vi "ReadEEPROMtoImage.vi"(8 "error in (no error)":errorcluster, 10 "Automation Refnum":refnum<k7>, 11 "IN":T1={"step name 1"="", "updata 2"="1000", "limitdata 3"="", "load vi name 4"="", "parameter 5"=""}) -> (0 "error out":errorcluster, 2 "reference out":refnum<k7>, 3 "Cluster":T2)   [LabVIEW 2013]
uses:
  Sub vi/Global constant.vi
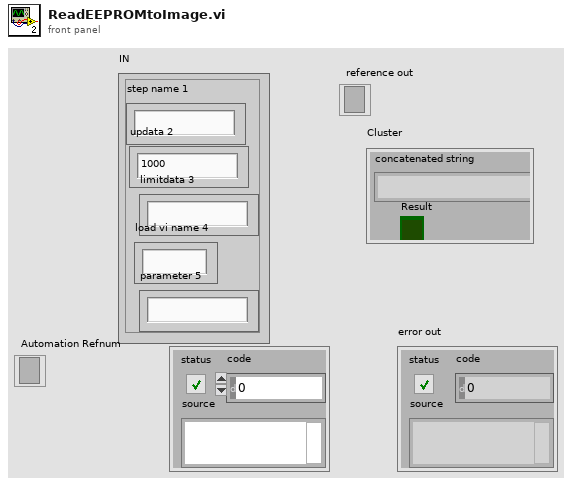
[diagram p1: front panel]
types:
  T1 = cluster{"step name 1":string, "updata 2":string, "limitdata 3":string, "load vi name 4":string, "parameter 5":string}
  T2 = cluster{"concatenated string":string, "Result":bool}
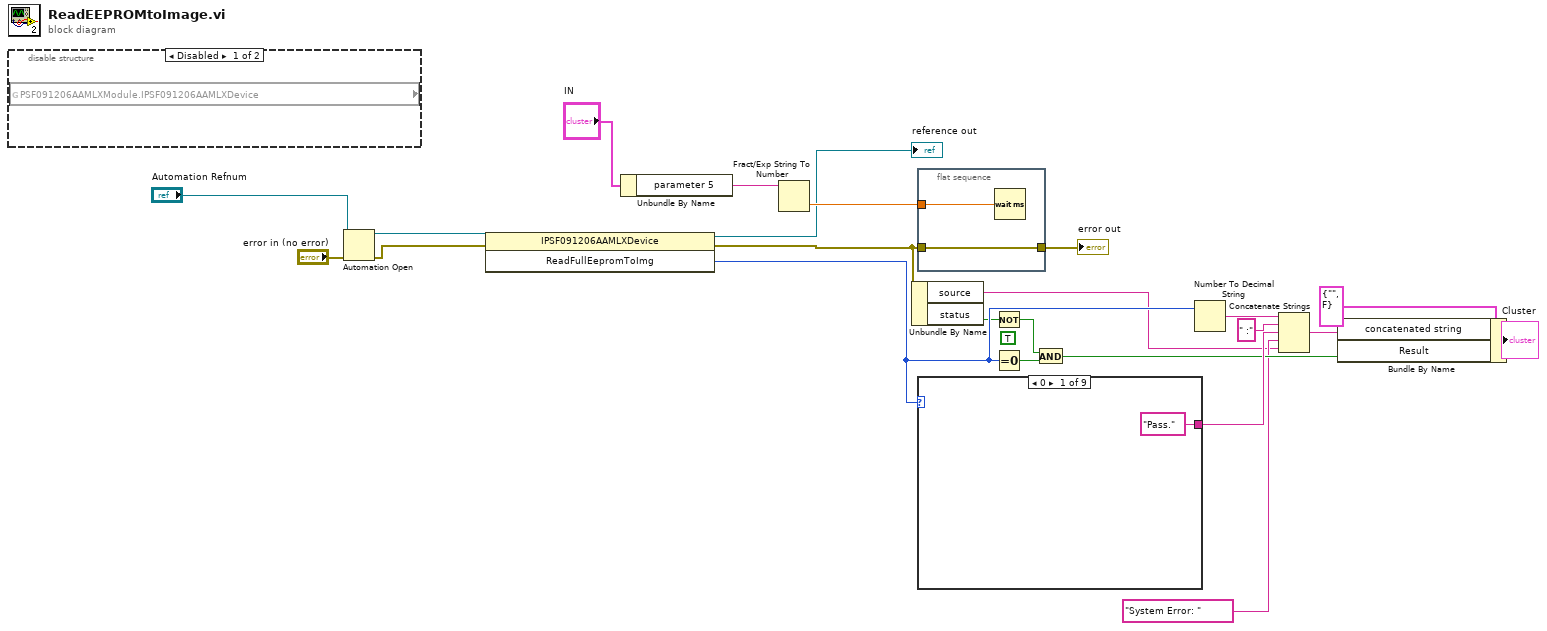
[diagram p0: block diagram]
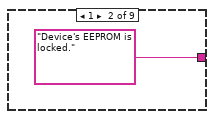
[diagram p3: hidden frame]
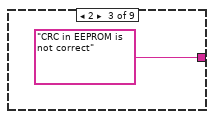
[diagram p4: hidden frame]
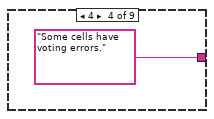
[diagram p5: hidden frame]
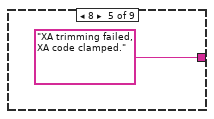
[diagram p6: hidden frame]
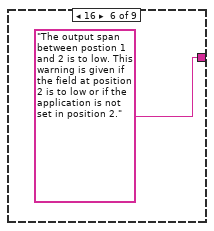
[diagram p7: hidden frame]
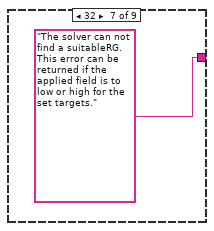
[diagram p8: hidden frame]
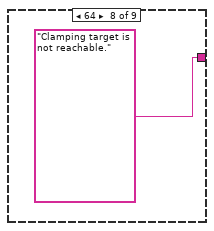
[diagram p9: hidden frame]
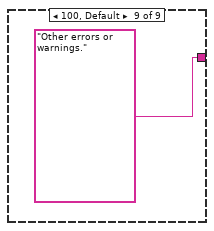
[diagram p10: hidden frame]
diagram:
  (unwired) TRUE
  n1 = disable-structure shown="Disabled" {
    frame Disabled {
      n2 = global read "Global constant.vi" "PSF091206AAMLXModule.IPSF091206AAMLXDevice"() -> ()  [unwired: 1 out]
    }
    frame Enabled {
    }
  }
  n3 = Automation Open(error in (no error)="error in (no error)", Automation Refnum="Automation Refnum") -> (Automation Refnum=w6:refnum<k7>, error out=w5:errorcluster)  [unwired: 2 in]
  n4 = invoke class="IPSF091206AAMLXDevice" method="ReadFullEepromToImg"(reference=w6, error in=w5) -> (reference out=→"reference out":refnum<k7>, error out=w11:errorcluster, "ReadFullEepromToImg"=w15:i32)  [unwired: 1 in]
  n5 = Unbundle By Name("IN") -> ("parameter 5"=w19:string)
  n6 = Fract/Exp String To Number(string=w19) -> (number=w20:dbl)  [unwired: 3 in, 1 out]
  n7 = Unbundle By Name(w11) -> ("source"=w4:string, "status"=w10:bool)
  n8 = flat-sequence {
    tunnel: w11 -> [w24]
    tunnel: w20 -> [w25]
    tunnel: [w24] -> w18
    frame #0 {
      n9 = Wait (ms)(milliseconds to wait=w25) -> ()  [unwired: 1 out]
    }
  }
  n10 = case shown="0" w15 {
    tunnel: ["Pass." "Device's EEPROM is locked." "CRC in EEPROM is not correct" "Some cells have voting errors." "XA trimming failed, XA code clamped." "The output span between postion 1 and 2 is to low. This warning is given if the field at position 2 is to low or if the application is not set in position 2." "The solver can not find a suitableRG. This error can be returned if the applied field is to low or high for the set targets." "Clamping target is not reachable." "Other errors or warnings."] -> w12
    frame 0 {
    }
    frame 1 {
    }
    frame 2 {
    }
    frame 4 {
    }
    frame 8 {
    }
    frame 16 {
    }
    frame 32 {
    }
    frame 64 {
    }
    frame 100, Default {
    }
  }
  n11 = Not(x=w10) -> (.not. x?=w3:bool)
  n12 = Equal To 0?(x=w15) -> (x = 0?=w9:bool)
  n13 = And(x=w3, y=w9) -> (x .and. y?=w8:bool)
  n14 = Number To Decimal String(number=w15) -> (decimal integer string=w14:string)  [unwired: 1 in]
  n15 = Concatenate Strings(w14, " :" ("string"), w12, "System Error: " ("string"), w4) -> (w16:string)
  n16 = Bundle By Name(cluster=T2 {"concatenated string"="", "Result"=FALSE} ("Cluster"), "concatenated string"=w16, "Result"=w8) -> (→"Cluster":T2)
  "error out" <- w18
